vi "FEA_Model_Particle-Node_Converter.vi"(7 "mode":T1(ring), 8 "Node":i32, 9 "Nodes":i32[](array[numeric]), 10 "Particle":i32, 11 "Particles":i32[](array[numeric])) -> (0 "Particle":i32, 1 "Particles":i32[](array[numeric]), 2 "Node":i32, 3 "Nodes":i32[](array[numeric]))   [LabVIEW 2021, in "FEA_Model.lvclass"]
uses:
  FEA_Model.lvclass
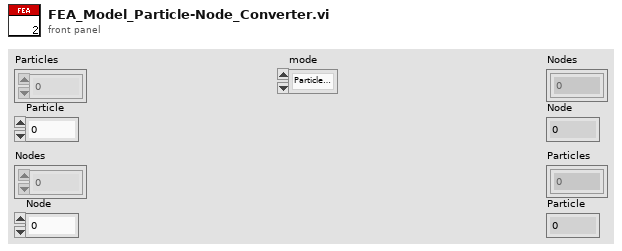
[diagram p1: front panel]
types:
  T1 = enum16{"Particles to Nodes", "Particle to Node", "Nodes to Particles", "Node to Particle"}
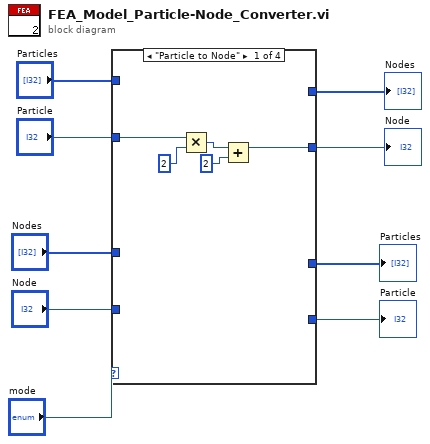
[diagram p0: block diagram]
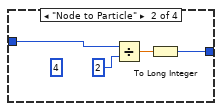
[diagram p2: hidden frame]
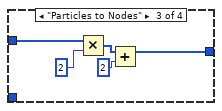
[diagram p3: hidden frame]
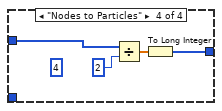
[diagram p4: hidden frame]
diagram:
  n1 = case shown="\"Particle to Node\"" "mode" {
    tunnel: "Particle" -> [w14 _ _ _]
    tunnel: "Particles" -> [_ _ w23 _]
    tunnel: [_ _ w20 _] -> w7
    tunnel: [w11 _ _ _] -> w6
    tunnel: "Node" -> [_ w15 _ _]
    tunnel: "Nodes" -> [_ _ _ w24]
    tunnel: [_ w16 _ _] -> w3
    tunnel: [_ _ _ w25] -> w2
    frame "Particle to Node" {
      n2 = Multiply(x=w14, y=2) -> (x*y=w12:i32)
      n3 = Add(x=w12, y=2) -> (x+y=w11:i32)
    }
    frame "Node to Particle" {
      (unwired) 4 ("y")
      n4 = Divide(x=w15, y=2) -> (x/y=w17:dbl)
      n5 = To Long Integer(number=w17) -> (32bit integer=w16:i32)
    }
    frame "Particles to Nodes" {
      n6 = Multiply(x=w23, y=2) -> (x*y=w21:i32[])
      n7 = Add(x=w21, y=2) -> (x+y=w20:i32[])
    }
    frame "Nodes to Particles" {
      (unwired) 4 ("y")
      n8 = Divide(x=w24, y=2) -> (x/y=w26:dbl[])
      n9 = To Long Integer(number=w26) -> (32bit integer=w25:i32[])
    }
  }
  "Nodes" <- w7
  "Node" <- w6
  "Particles" <- w2
  "Particle" <- w3
